vi "ClimbQCP.vi"   [LabVIEW 2017]
uses:
  <userlib>/836-Library/System/QCP_V2/QCPSupportCode/QCP_GetDbl.vi
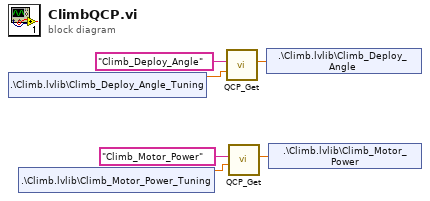
[diagram p0: block diagram]
diagram:
  n1 = shared-variable ".\\Climb.lvlib\\Climb_Deploy_Angle_Tuning"() -> (w2:dbl)  [unwired: 1 in, 1 out]
  n2 = shared-variable ".\\Climb.lvlib\\Climb_Motor_Power_Tuning"() -> (w1:dbl)  [unwired: 1 in, 1 out]
  n3 = call-poly <userlib>:"QCP_Get.vi"("Tuning Value"=w2, "Value Name"="Climb_Deploy_Angle") -> ("Value"=w5:dbl)  [unwired: 7 in, 2 out]
  n4 = call-poly <userlib>:"QCP_Get.vi"("Tuning Value"=w1, "Value Name"="Climb_Motor_Power") -> ("Value"=w6:dbl)  [unwired: 7 in, 2 out]
  n5 = shared-variable ".\\Climb.lvlib\\Climb_Deploy_Angle"(w5) -> ()  [unwired: 1 in, 1 out]
  n6 = shared-variable ".\\Climb.lvlib\\Climb_Motor_Power"(w6) -> ()  [unwired: 1 in, 1 out]
